vi "Tusk.Create.vi"(7 "This VI":refnum<vi>, 11 "Tusk in":refnum<class "Tusk.lvclass">) -> (0 "error out":errorcluster, 4 "Tusk out":refnum<class "Tusk.lvclass">, 6 "error out (copy)":errorcluster)   [LabVIEW 2018, in "Application.lvlib" / "Tusk.lvclass"]
uses:
  Tusk.lvclass
  Store Class/Store.lvclass/Store.ctl
  Tusk.lvclass/Tusk.ctl
  Controls/Tusk.TuskBoxOperation.ctl
  <vilib>/Utility/error.llb/Error Cluster From Error Code.vi
  Store Class/Store.lvclass
  Dictionary Class/Dictionary.lvclass
  <vilib>/ErrorRing/Error Ring.xnode
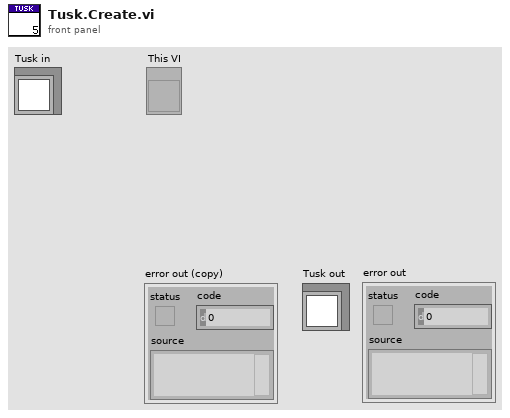
[diagram p1: front panel]
types:
  T1 = typedef "Application.lvlib/Tusk.lvclass/Tusk.TuskBoxOperation.ctl" = enum16{"Add", "Get", "Remove"}
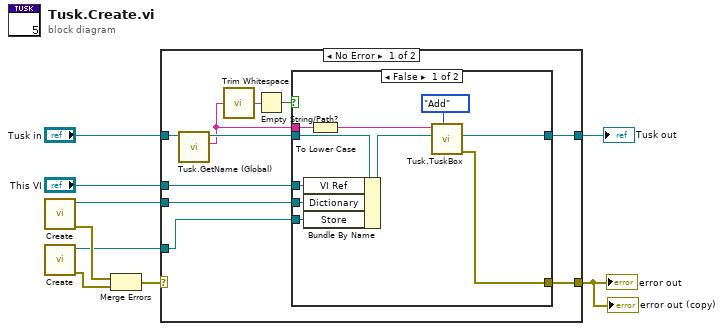
[diagram p0: block diagram]
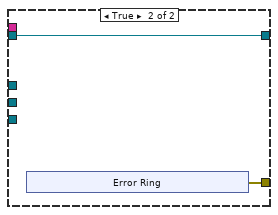
[diagram p2: hidden frame]
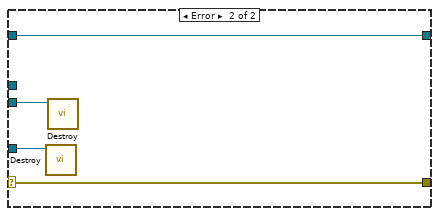
[diagram p3: hidden frame]
diagram:
  n1 = call "Create.vi"() -> ("error out"=w8:errorcluster, "Dictionary out"=w4:refnum<class "Dictionary.lvclass">)  [unwired: 10 in]
  n2 = call "Create.vi"() -> ("error out"=w7:errorcluster, "Store out"=w5:refnum<class "Store.lvclass">)  [unwired: 10 in]
  n3 = Merge Errors(w8, w7) -> (w6:errorcluster)
  n4 = case shown="No Error" w6 {
    selector: w6 -> [_ w40]
    tunnel: [w16 w37] -> w9
    tunnel: [w15 w40] -> w1
    tunnel: w5 -> [w18 w38]
    tunnel: w4 -> [w19 w39]
    tunnel: "Tusk in" -> [w14 w37]
    tunnel: "This VI" -> [w17 _]
    frame No Error {
      n5 = call "Tusk.GetName (Global).vi"("Tusk in"=w14) -> ("Name(Global)"=w12:string, "Tusk out"=w13:refnum<class "Tusk.lvclass">)  [unwired: 8 in, 1 out]
      n6 = call <vilib>:"Trim Whitespace.vi"("string"=w12) -> ("trimmed string"=w11:string)  [unwired: 1 in]
      n7 = Empty String/Path?(string/path=w11) -> (empty?=w10:bool)
      n8 = case shown="False" w10 {
        tunnel: w19 -> [w29 _]
        tunnel: w18 -> [w28 _]
        tunnel: w17 -> [w27 _]
        tunnel: [w25 w31] -> w16
        tunnel: [w22 w30] -> w15
        tunnel: w13 -> [w21 w31]
        tunnel: w12 -> [w20 _]
        frame False {
          n9 = Bundle By Name(cluster=w21, "VI Ref"=w27, "Dictionary"=w29, "Store"=w28) -> (w26:refnum<class "Tusk.lvclass">)
          n10 = To Lower Case(string=w20) -> (all lower case string=w23:string)
          n11 = call "Tusk.TuskBox.vi"("Operation"=Tusk.TuskBoxOperation."Add", "Tusk in"=w26, "Global Name"=w23) -> ("error out"=w22:errorcluster, "Tusk out"=w25:refnum<class "Tusk.lvclass">)  [unwired: 7 in]
        }
        frame True {
          n12 = xnode "Error Ring"() -> ("error out"=w30:errorcluster)
        }
      }
    }
    frame Error {
      n13 = call "Destroy.vi"("Store in"=w38) -> ()  [unwired: 10 in, 1 out]
      n14 = call "Destroy.vi"("Dictionary in"=w39) -> ()  [unwired: 8 in, 3 out]
    }
  }
  "error out (copy)" <- w1
  "Tusk out" <- w9
  "error out" <- w1
